vi "kepcoScanStandAloneHostTest.vi"() -> ()   [LabVIEW 2014]
uses:
  <vilib>/rvi/interface/nirviOpenFPGA/nirviOpenFPGA.xnode
  <vilib>/rvi/interface/nirviReadWriteControl/nirviReadWriteControl.xnode
  <vilib>/rvi/interface/Simulation/niFpgaSimulationCallBeginRW.vi
  <vilib>/rvi/errors/niLvFpgaAdjustHostInterfaceError.vi
  <vilib>/rvi/interface/nirviMethod/nirviMethod.xnode
  <vilib>/rvi/interface/nirviCloseFPGA/nirviCloseFPGA.xnode
  <vilib>/FPGAPlugInAG/Dynamic/niLvFpga_Reset_Dynamic.vi
  <vilib>/FPGAPlugInAG/Dynamic/niLvFpga_Run_Dynamic.vi
  FPGA Bitfiles/TiTaProj_DAF_kepcoScanStandAlone.lvbitx
  <vilib>/rvi/errors/niLvFpgaMergeErrorWithErrorCode.vi
  <vilib>/FPGAPlugInAG/Dynamic/niLvFpga_ReadFifo_Dynamic.vi
  <vilib>/FPGAPlugInAG/PXI-7852R/niLvFpga_Open_PXI-7852R.vi
  <vilib>/rvi/interface/common/dynamic/niFpgaDynamicAddResources.vi
  <vilib>/FPGAPlugInAG/Dynamic/niLvFpga_WriteFifo_Dynamic.vi
  <vilib>/FPGAPlugInAG/Dynamic/niLvFpga_Close_Dynamic.vi
panel:
  out "actStep":i32
  out "actTrack":i32
  out "stepSize(V)":dbl format="%#.20f"
  in  "VRefn":dbl
  in  "VRefp":dbl
  out "nOfSteps":i32
  in  "SetValuesforNextScan":bool=TRUE
  in  "invertInOddnOfTrack":bool
  out "i outer":i32
  in  "waitAfterReset(25nsTicks)":u16
  in  "Go":bool
  in  "abort":bool
  out "timeoutDAC":bool
  in  "Data":i32[](array[numeric])=[65536, 1048576, 4, 3, 32768, 1572864, 5, 2, 16384, 1310720, 6, 2] format="%024b"
  in  "nOfScanRegions":i32=1
  in  "waitForKepco(25nsTicks)":u16=1
  in  "waitForDmm(25nsTicks)":u32=1
  # "Each  scan region consists of: [step, start, nOfSteps, nOfTracks]"
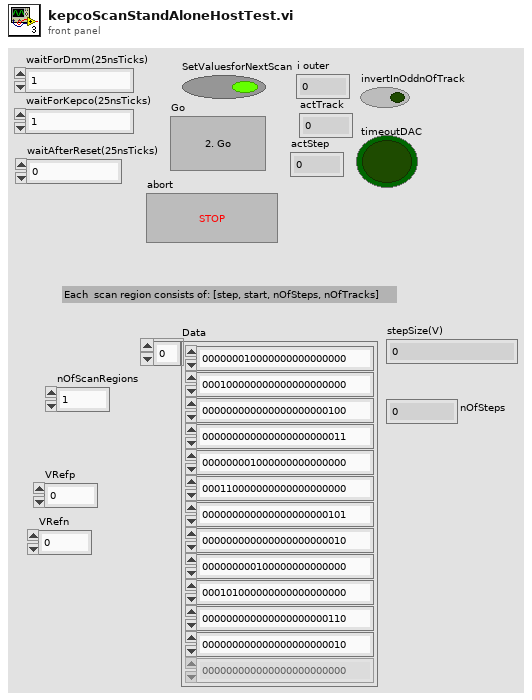
[diagram p1: front panel]
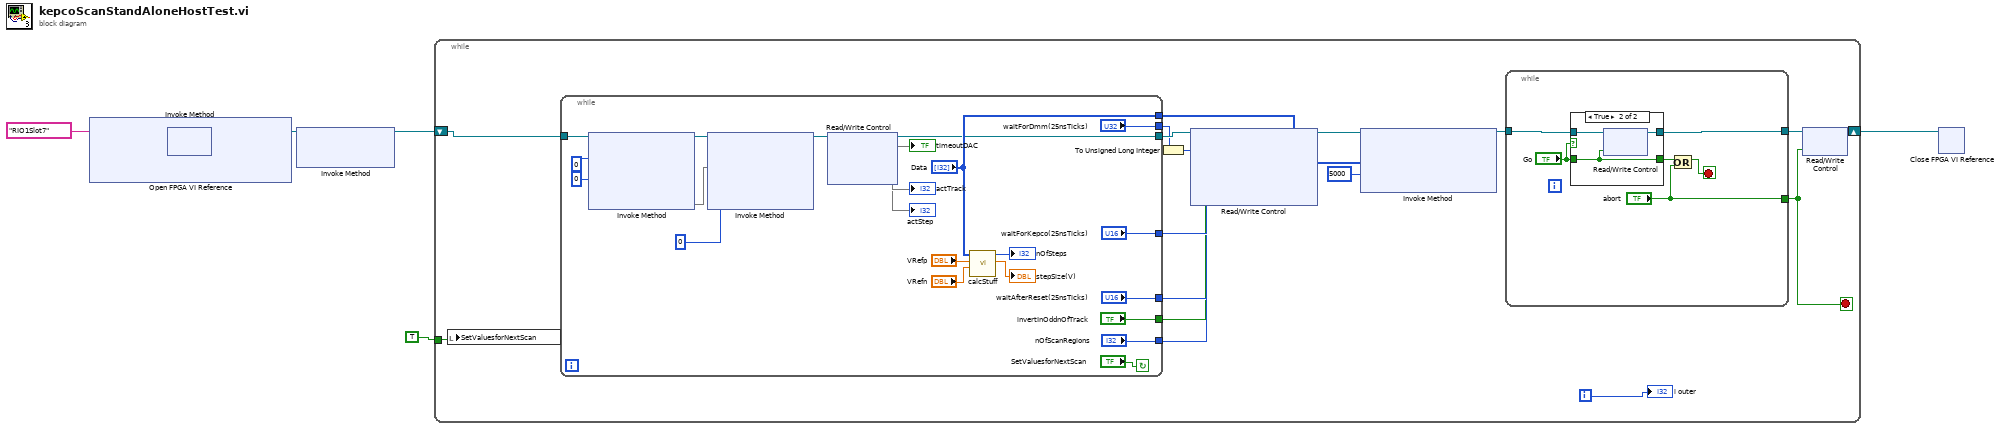
[diagram p0: block diagram]
diagram:
  n1 = xnode ("Open FPGA VI Reference")("resource name"=tag "RIO1Slot7") -> ("FPGA VI Reference Out"=w6:refnum<k20>)  [unwired: 1 in, 1 out]
  n2 = xnode "Invoke Method"("FPGA VI Reference In"=w6) -> ("FPGA VI Reference Out"=w2:refnum<k20>)  [unwired: 1 in, 1 out]
  n3 = xnode "Invoke Method"("FPGA VI Reference In"=w2) -> ("FPGA VI Reference Out"=w1:refnum<k20>)  [unwired: 2 in, 1 out]
  n4 = while {
    shift-right: [w18] -> w5
    shift-left: w1 -> [w15]
    tunnel: TRUE ("SetValuesforNextScan") -> [w13]
    i -> [w17]
    stop <- w16 stop-if-true
    n5 = local write "SetValuesforNextScan"(w13) -> ()
    n6 = while {
      tunnel: w15 -> [w45]
      tunnel: [w33] -> w14
      tunnel: ["waitForDmm(25nsTicks)"] -> w12
      tunnel: ["waitForKepco(25nsTicks)"] -> w11
      tunnel: ["nOfScanRegions"] -> w10
      tunnel: ["waitAfterReset(25nsTicks)"] -> w9
      tunnel: ["invertInOddnOfTrack"] -> w8
      tunnel: ["Data"] -> w7
      stop <- "SetValuesforNextScan" continue-if-true
      n7 = xnode "Invoke Method"("FPGA VI Reference In"=w45, "Number of Elements"=u32 0, "Timeout (ms)"=0) -> ("FPGA VI Reference Out"=w29:refnum<k20>, "Elements Remaining"=w25)  [unwired: 1 in, 2 out]
      n8 = xnode "Invoke Method"("FPGA VI Reference In"=w29, "Number of Elements"=w25, "Timeout (ms)"=0) -> ("FPGA VI Reference Out"=w26:refnum<k20>)  [unwired: 1 in, 3 out]
      n9 = xnode "Read/Write Control"("FPGA VI Reference In"=w26) -> ("FPGA VI Reference Out"=w33:refnum<k20>, "timeoutDAC"=→"timeoutDAC", "actTrack"=→"actTrack", "actStep"=→"actStep")  [unwired: 1 in, 1 out]
      n10 = call "calcStuff.vi"("VRefn"="VRefn", "VRefp"="VRefp", "Data"="Data") -> ("stepSize(V)"=→"stepSize(V)":dbl, "nOfSteps"=→"nOfSteps":i32)  [unwired: 7 in]
    }
    n11 = To Unsigned Long Integer(number=w12) -> (unsigned 32bit integer=w22:u32)
    n12 = xnode "Read/Write Control"("FPGA VI Reference In"=w14, "waitForDmm(25nsTicks)"=w22, "waitForKepco(25nsTicks)"=w11, "nOfScanRegions"=w10, "waitAfterReset(25nsTicks)"=w9, "invertInOddnOfTrack"=w8) -> ("FPGA VI Reference Out"=w21:refnum<k20>)  [unwired: 1 in, 1 out]
    n13 = xnode "Invoke Method"("FPGA VI Reference In"=w21, "Data"=w7, "Timeout (ms)"=5000) -> ("FPGA VI Reference Out"=w19:refnum<k20>)  [unwired: 1 in, 2 out]
    n14 = while {
      tunnel: w19 -> [w51]
      tunnel: [w46] -> w23
      tunnel: ["abort"] -> w16
      stop <- w48 stop-if-true
      n15 = case shown="True" "Go" {
        tunnel: w51 -> [w53 w56]
        tunnel: [w53 w55] -> w46
        tunnel: "Go" -> [w52 w54]
        tunnel: [w52 w54] -> w49
        frame False {
        }
        frame True {
          n16 = xnode "Read/Write Control"("FPGA VI Reference In"=w56, "Go"=w54) -> ("FPGA VI Reference Out"=w55:refnum<k20>)  [unwired: 1 in, 1 out]
        }
      }
      n17 = Or(x=w49, y="abort") -> (x .or. y?=w48:bool)
    }
    n18 = xnode "Read/Write Control"("FPGA VI Reference In"=w23, "abort"=w16) -> ("FPGA VI Reference Out"=w18:refnum<k20>)  [unwired: 1 in, 1 out]
    "i outer" <- w17
  }
  n19 = xnode "Close FPGA VI Reference"("FPGA VI Reference In"=w5) -> ()  [unwired: 1 in, 1 out]
